vi "Element Init.vi"(7 "VolatusAPI":refnum<class "VolatusAPI.lvclass">, 8 "error in (no error)":errorcluster, 10 "JSON":string, 11 "LoggingControl in":refnum<class "GroupLoggingControl.lvclass">) -> (0 "error out":errorcluster, 3 "LoggingControl out":refnum<class "GroupLoggingControl.lvclass">)   [LabVIEW 2020, in "VolatusGUIElements.lvlib" / "GroupLoggingControl.lvclass"]
uses:
  GroupLoggingControl.lvclass
  C:/dev/lv20CE/relink/lv-volatus/VolatusGUI/GUI Element/GUI Element.lvclass
  Volatus/VolatusAPI/VolatusAPI.lvclass
  JSON.ctl
  Prompt Result.ctl
  Prompt Action.ctl
  Status.ctl
  Log Group.ctl
  Log Group Status.ctl
  Command Info.ctl
  lv-vecto/Vecto/Channel STR/Channel STR.lvclass
  Target Info.ctl
  VolatusGUI/GUI Element/GUI Element.lvclass/GUI Element.ctl
  GroupLoggingControl.lvclass/GroupLoggingControl.ctl
  6b4406ff-dbb0-478f-9794-4f2464f74e8d.vi
  <vilib>/JDP Science/JSONtext/JSON text to Variant.vi
  <vilib>/JDP Science/JSONtext/LVClass Serializer/JSONtext LVClass Serializer.lvclass
  VolatusGUI/GUI Element/GUI Element.lvclass
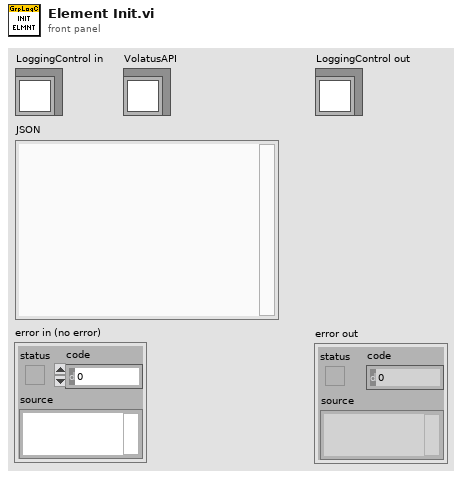
[diagram p1: front panel]
types:
  T1 = typedef "VolatusGUIElements.lvlib/GroupLoggingControl.lvclass/Status.ctl" = cluster{"Groups":T2[], "Targets":T5[]}
  T2 = typedef "VolatusGUIElements.lvlib/GroupLoggingControl.lvclass/Log Group.ctl" = cluster{"Status":T3, "Command Info":T4, "State":refnum<class "Channel STR.lvclass">, "Logging":bool}
  T3 = typedef "VolatusGUIElements.lvlib/GroupLoggingControl.lvclass/Log Group Status.ctl" = cluster{"Group":string, "Group Color":u32, "Button":bool}
  T4 = typedef "VolatusGUIElements.lvlib/GroupLoggingControl.lvclass/Command Info.ctl" = cluster{"Commanding":bool, "Cmd Time":dbl, "Group ID":string}
  T5 = typedef "VolatusGUIElements.lvlib/GroupLoggingControl.lvclass/Target Info.ctl" = cluster{"Node":string, "Node Color":u32, "Groups":T2[]}
  T6 = typedef "VolatusGUIElements.lvlib/GroupLoggingControl.lvclass/Prompt Result.ctl" = cluster{"Action":T7, "Series":string, "Timestamp":string, "Target (All)":string, "Group (All)":string}
  T7 = typedef "VolatusGUIElements.lvlib/GroupLoggingControl.lvclass/Prompt Action.ctl" = enum16{"Cancelled", "Started"}
  T8 = typedef "VolatusGUIElements.lvlib/GroupLoggingControl.lvclass/JSON.ctl" = cluster{"Groups":cluster{"Label":string, "Group":string}[], "Targets":cluster{"Node":string, "Groups":cluster{"Label":string, "Group":string}[]}[]}
  T9 = cluster{"Node":string, "Groups":cluster{"Label":string, "Group":string}[]}[]
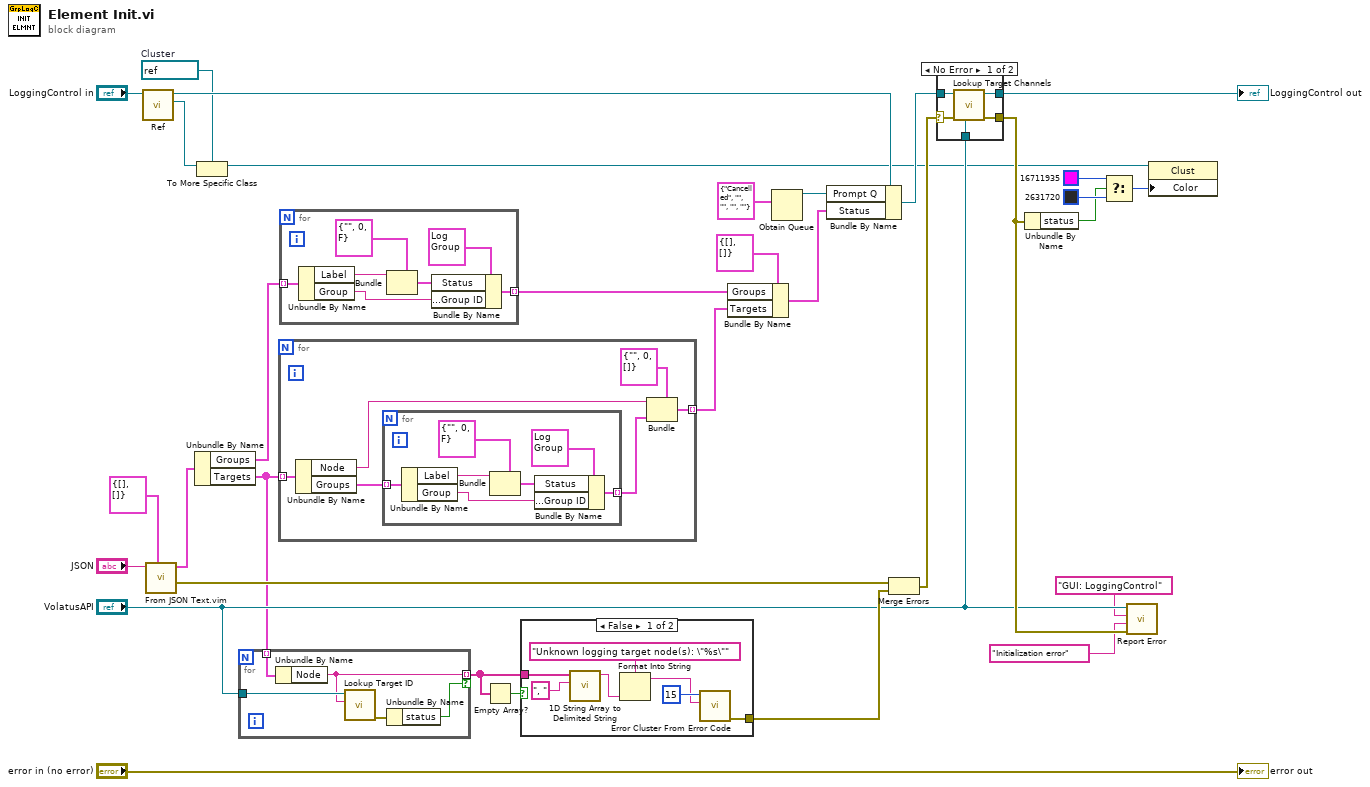
[diagram p0: block diagram]
diagram:
  w9 = refnum<vi> refnum  # Cluster
  n1 = call "Ref.vi"("GUI Element in"="LoggingControl in") -> ("Ref"=w10:refnum<vi>, "GUI Element out"=w11:refnum<class "GroupLoggingControl.lvclass">)  [unwired: 9 in]
  n2 = call "From JSON Text.vim"("Data Type and Default Value"=T8 {"Groups"=[], "Targets"=[]} ("JSON"), "JSON"="JSON") -> ("error out"=w26:errorcluster, "Data out"=w27:T8)  [unwired: 8 in]
  n3 = Unbundle By Name(w27) -> ("Groups"=w3:cluster{"Label":string, "Group":string}[], "Targets"=w6:T9)
  n4 = To More Specific Class(target class=w9, reference=w10) -> (specific class reference=w8:refnum<vi>)  [unwired: 1 in, 1 out]
  n5 = for {
    tunnel: "VolatusAPI" -> [w37]
    tunnel: w6 -> [w34] mode=indexing
    tunnel: [w33] -> w24 mode=indexing if=w35
    n6 = Unbundle By Name(w34) -> ("Node"=w33:string)
    n7 = call "Lookup Target ID.vi"("Target Name"=w33, "VolatusAPI in"=w37) -> ("error out"=w36:errorcluster)  [unwired: 6 in, 3 out]
    n8 = Unbundle By Name(w36) -> ("status"=w35:bool)
  }
  n9 = for {
    tunnel: w6 -> [w43] mode=indexing
    tunnel: [w38] -> w4 mode=indexing
    n10 = Unbundle By Name(w43) -> ("Node"=w42:string, "Groups"=w40:cluster{"Label":string, "Group":string}[])
    n11 = for {
      tunnel: w40 -> [w50] mode=indexing
      tunnel: [w45] -> w39 mode=indexing
      n12 = Unbundle By Name(w50) -> ("Label"=w49:string, "Group"=w44:string)
      n13 = Bundle(cluster=T3 {"Group"="", "Group Color"=0, "Button"=FALSE} ("Log Group Status"), "Group"=w49) -> (w46:T3)  [unwired: 2 in]
      n14 = Bundle By Name(cluster=T2 {"Status"={"Group"="", "Group Color"=0, "Button"=FALSE}, "Command Info"={"Commanding"=FALSE, "Cmd Time"=0.0, "Group ID"=""}, "State"=refnum, "Logging"=FALSE} ("Log Group"), "Status"=w46, "Command Info.Group ID"=w44) -> (w45:T2)
    }
    n15 = Bundle(cluster=T5 {"Node"="", "Node Color"=0, "Groups"=[]} ("Node Info"), "Node"=w42, "Groups"=w39) -> (w38:T5)  [unwired: 1 in]
  }
  n16 = for {
    tunnel: w3 -> [w57] mode=indexing
    tunnel: [w52] -> w2 mode=indexing
    n17 = Unbundle By Name(w57) -> ("Label"=w56:string, "Group"=w51:string)
    n18 = Bundle(cluster=T3 {"Group"="", "Group Color"=0, "Button"=FALSE} ("Log Group Status"), "Group"=w56) -> (w53:T3)  [unwired: 2 in]
    n19 = Bundle By Name(cluster=T2 {"Status"={"Group"="", "Group Color"=0, "Button"=FALSE}, "Command Info"={"Commanding"=FALSE, "Cmd Time"=0.0, "Group ID"=""}, "State"=refnum, "Logging"=FALSE} ("Log Group"), "Status"=w53, "Command Info.Group ID"=w51) -> (w52:T2)
  }
  n20 = Empty Array?(array=w24) -> (empty?=w25:bool)
  n21 = case shown="False" w25 {
    tunnel: w24 -> [w64 _]
    tunnel: [w58 _] -> w23
    frame False {
      n22 = call <vilib>:"1D String Array to Delimited String.vi"("delimiter"=", ", "string array"=w64) -> ("delimited string"=w61:string)  [unwired: 9 in]
      n23 = Format Into String(format string="Unknown logging target node(s): \"%s\"", w61) -> (resulting string=w59:string)  [unwired: 2 in, 1 out]
      n24 = call <vilib>:"Error Cluster From Error Code.vi"("error message (\"\")"=w59, "error code (0)"=15) -> ("error out"=w58:errorcluster)  [unwired: 7 in]
    }
    frame True {
    }
  }
  n25 = Bundle By Name(cluster=T1 {"Groups"=[], "Targets"=[]} ("Status"), "Groups"=w2, "Targets"=w4) -> (w1:T1)
  n26 = Obtain Queue(element data type=T6 {"Action"=enum."Cancelled", "Series"="", "Timestamp"="", "Target (All)"="", "Group (All)"=""} ("Prompt Result")) -> (queue out=w12:refnum<queue>)  [unwired: 4 in, 2 out]
  n27 = Bundle By Name(cluster=w11, "Prompt Q"=w12, "Status"=w1) -> (w30:refnum<class "GroupLoggingControl.lvclass">)
  n28 = Merge Errors(w26, w23) -> (w15:errorcluster)
  n29 = case shown="No Error" w15 {
    selector: w15 -> [w67 w71]
    tunnel: w30 -> [w69 w70]
    tunnel: [w68 w70] -> w16
    tunnel: [w66 w71] -> w32
    tunnel: "VolatusAPI" -> [w65 _]
    frame No Error {
      n30 = call "Lookup Target Channels.vi"("VolatusAPI"=w65, "error in (no error)"=w67, "LoggingControl in"=w69) -> ("error out"=w66:errorcluster, "LoggingControl out"=w68:refnum<class "GroupLoggingControl.lvclass">)  [unwired: 7 in]
    }
    frame Error {
    }
  }
  "LoggingControl out" <- w16
  n31 = Unbundle By Name(w32) -> ("status"=w18:bool)
  n32 = Select(t=u32 16711935 ("Color"), s=w18, f=u32 2631720 ("Color")) -> (s? t:f=w19:u32)
  n33 = call "Report Error.vi"("error in (no error)"=w32, "Message"="Initialization error", "Context"="GUI: LoggingControl", "VolatusAPI in"="VolatusAPI") -> ()  [unwired: 6 in, 2 out]
  n34 = property class="Clust"(reference=w8, "Color"=w19) -> ()  [unwired: 1 in, 2 out]
  "error out" <- "error in (no error)"
